vi "Get User Filename and Path.vi"(8 "error in (no error)":errorcluster) -> (0 "error out":errorcluster, 2 "TXT File Path":path, 3 "CSV File Path":path)   [LabVIEW 2016]
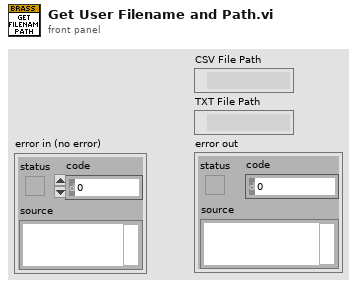
[diagram p1: front panel]
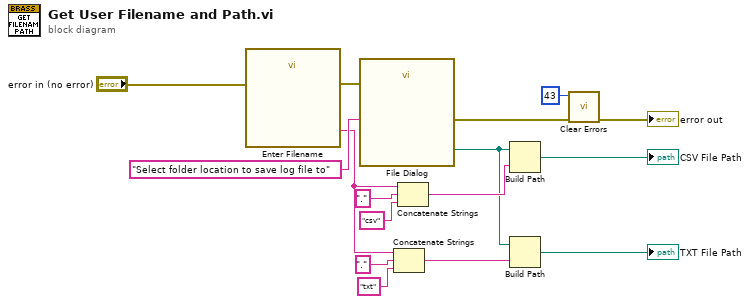
[diagram p0: block diagram]
diagram:
  n1 = call "Enter Filename"("error in (no error)"="error in (no error)") -> ("Filename"=w5:string, "error out"=w16:errorcluster)  [unwired: 16 in, 1 out]
  n2 = call "File Dialog"("prompt"="Select folder location to save log file to", "error in"=w16) -> ("selected path"=w6:path, "error out"=w3:errorcluster)  [unwired: 10 in, 2 out]
  n3 = Concatenate Strings(w5, "." ("string"), "txt" ("string")) -> (w9:string)
  n4 = Concatenate Strings(w5, "." ("string"), "csv" ("string")) -> (w12:string)
  n5 = Build Path(base path=w6, name or relative path=w12) -> (appended path=→"CSV File Path":path)
  n6 = Build Path(base path=w6, name or relative path=w9) -> (appended path=→"TXT File Path":path)
  n7 = call <vilib>:"Clear Errors.vi"("error in (no error)"=w3, "specific error code to clear (0: all)"=43) -> ("error out"=→"error out":errorcluster)  [unwired: 4 in, 1 out]
